vi "Start Live Mode.vi"(7 "Correlation ID":u32, 8 "error in (no error)":errorcluster, 9 "Mode":T1=enum."Live", 10 "Camera Settings":T2={"Exposure Time (ms)"=100.0, "Binning"=enum."2x2", "Scan Mode"=0, "Frames to Acquire"=1000.0, "Pixel Correction"=FALSE, "Frames to Skip"=0, "File Path"=path "", "Duty cycle"=0.0, "ALEX"=FALSE, "Shutter Enable"=[], "fluidics trigger, ms (0=disabled)"=0.0, "Bit Depth"=16, "Image Width (px)"=0, "Image Height (px)"=0, "Horizontal Offset (px)"=0, "Vertical Offset (px)"=0} {"fluidics trigger, ms (0=disabled)" max=60000.0 step=1.0; "Exposure Time (ms)" min=1.0 max=10000.0 step=1.0}, 11 "Application in":refnum<class "Application.lvclass">) -> (0 "error out":errorcluster, 3 "Application out":refnum<class "Application.lvclass">)   [LabVIEW 2023, in "Application.lvlib" / "Application.lvclass"]
uses:
  Application.lvclass
  Resources/Type Defs/Camera Settings.ctl
  Mode.ctl
  Application.lvclass/Application.ctl
  Hardware/Camera Messages/Start Live Mode Msg/Start Live Mode Msg.lvclass/Start Live Mode Msg.ctl
  <vilib>/ActorFramework/Message Enqueuer/Message Enqueuer.lvclass/Message Enqueuer.ctl
  Hardware/Sync Device Messages/Start Streaming Msg/Start Streaming Msg.lvclass/Start Streaming Msg.ctl
  <vilib>/ActorFramework/Message Enqueuer/Enqueue.vi
  Hardware/Camera Messages/Start Live Mode Msg/Start Live Mode Msg.lvclass
  Hardware/Sync Device Messages/Start Streaming Msg/Start Streaming Msg.lvclass
  Resources/GLOBAL/GLOBAL Time-critical.vi
  <vilib>/ActorFramework/Message Priority Queue/Priority Enqueue.vi
  Application.lvlib
  Hardware/NI DAQ/NI DAQ.lvlib
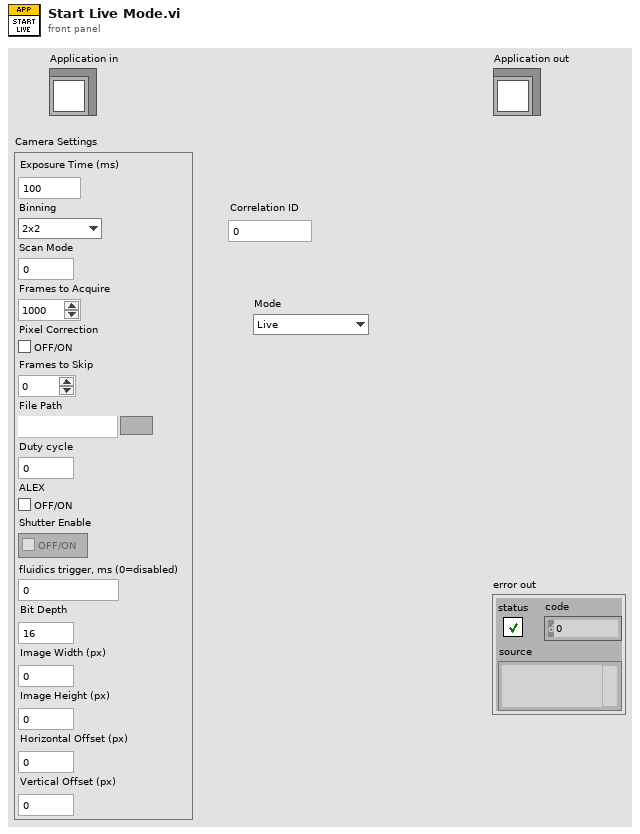
[diagram p1: front panel]
types:
  T1 = typedef "Application.lvlib/Mode.ctl" = enum16{"Idle", "Cancel", "Live", "Stream", "Autofocus", "Z-Stack", "Montage", "Saving", "Stage Scan", "Laser Adjust"}
  T2 = typedef "Camera Settings.ctl" = cluster{"Exposure Time (ms)":dbl, "Binning":enum16{"1x1", "2x2", "4x4"}, "Scan Mode":i32, "Frames to Acquire":dbl, "Pixel Correction":bool, "Frames to Skip":u32, "File Path":path, "Duty cycle":dbl, "ALEX":bool, "Shutter Enable":bool[], "fluidics trigger, ms (0=disabled)":dbl, "Bit Depth":u16, "Image Width (px)":u16, "Image Height (px)":u16, "Horizontal Offset (px)":u16, "Vertical Offset (px)":u16}
  T3 = typedef "Shutter Configuration.ctl" = cluster{"IO Line":tag, "Name":string, "Wavelength":u16, "Max rate (Hz)":dbl}
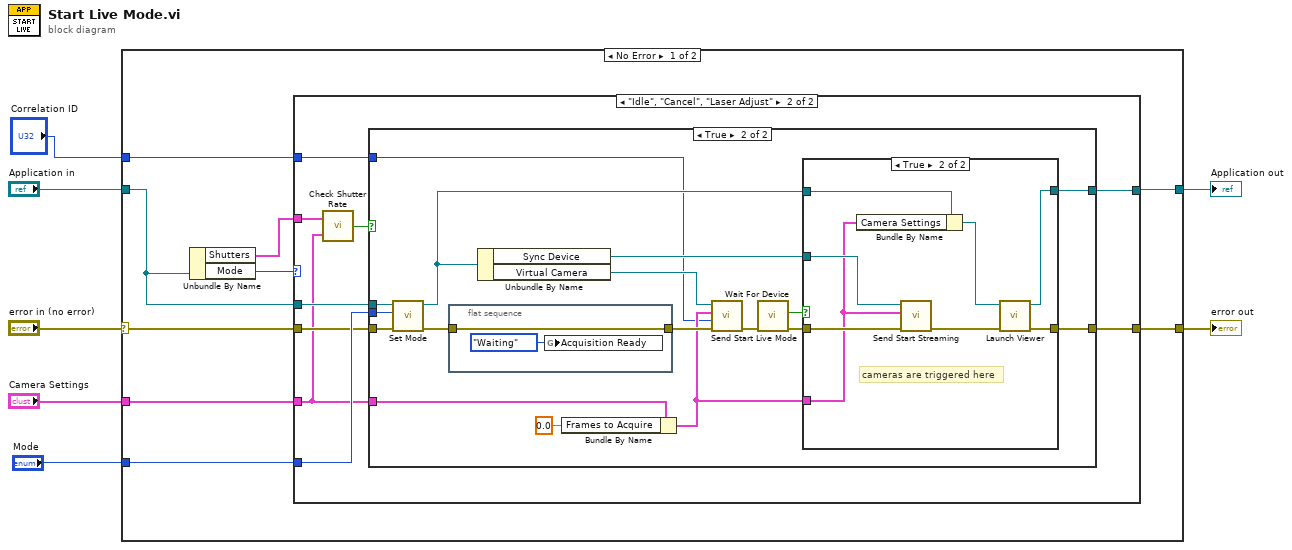
[diagram p0: block diagram]
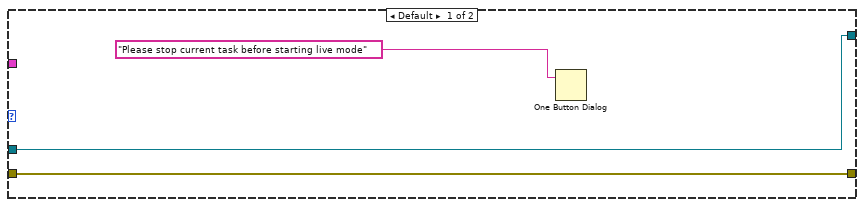
[diagram p2: hidden frame]
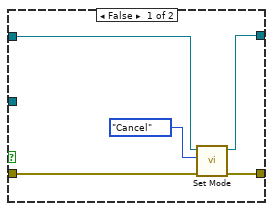
[diagram p4: hidden frame]
diagram:
  n1 = case shown="No Error" "error in (no error)" {
    selector: "error in (no error)" -> [w13 w64]
    tunnel: [w16 w64] -> w6
    tunnel: [w15 w63] -> w4
    tunnel: "Application in" -> [w12 w63]
    tunnel: "Camera Settings" -> [w14 _]
    tunnel: "Mode" -> [w10 _]
    tunnel: "Correlation ID" -> [w8 _]
    frame No Error {
      n2 = Unbundle By Name(w12) -> ("Shutters"=w9:T3[], "Mode"=w11:T1)
      n3 = case shown="\"Idle\", \"Cancel\", \"Laser Adjust\"" w11 {
        tunnel: [w18 w25] -> w16
        tunnel: [w19 w24] -> w15
        tunnel: w14 -> [_ w23]
        tunnel: w13 -> [w18 w27]
        tunnel: w12 -> [w19 w26]
        tunnel: w10 -> [_ w28]
        tunnel: w9 -> [_ w22]
        tunnel: w8 -> [_ w20]
        frame Default {
          n4 = One Button Dialog(message="Please stop current task before starting live mode") -> ()  [unwired: 1 in, 1 out]
        }
        frame "Idle", "Cancel", "Laser Adjust" {
          n5 = call "Check Shutter Rate.vi"("Camera Settings"=w23, "Shutters"=w22) -> ("OK?"=w21:bool)
          n6 = case shown="True" w21 {
            tunnel: w28 -> [_ w46]
            tunnel: w27 -> [w29 w45]
            tunnel: w26 -> [w30 w44]
            tunnel: [w29 w41] -> w25
            tunnel: [w30 w40] -> w24
            tunnel: w23 -> [_ w33]
            tunnel: w20 -> [_ w31]
            frame False {
            }
            frame True {
              n7 = call-dynamic "Set Mode.vi"("error in (no error)"=w45, "New Mode"=w46, "Application in"=w44) -> ("error out"=w43:errorcluster, "Application out"=w42:refnum<class "Application.lvclass">)  [unwired: 7 in]
              n8 = flat-sequence {
                tunnel: w43 -> [w62]
                tunnel: [w62] -> w39
                frame #0 {
                  n9 = global write "GLOBAL Time-critical.vi" "Acquisition Ready"(enum16{"Waiting", "Ready", "Fail", "Timeout"}."Waiting" ("Acquisition Ready")) -> ()
                }
              }
              n10 = Unbundle By Name(w42) -> ("Sync Device"=w47:refnum<class "Message Enqueuer.lvclass">, "Virtual Camera"=w38:refnum<class "Message Enqueuer.lvclass">)
              n11 = Bundle By Name(cluster=w33, "Frames to Acquire"=0.0) -> (w32:T2)
              n12 = call "Send Start Live Mode.vi"("error in (no error)"=w39, "Correlation ID"=w31, "Camera Settings"=w32, "Message Enqueuer"=w38) -> ("error out"=w37:errorcluster)  [unwired: 6 in, 1 out]
              n13 = call "Wait For Device.vi"("error in"=w37) -> ("error out"=w35:errorcluster, "Success?"=w36:bool)  [unwired: 9 in]
              n14 = case shown="True" w36 {
                tunnel: w47 -> [_ w54]
                tunnel: w42 -> [w51 w60]
                tunnel: [w49 w59] -> w41
                tunnel: [w50 w58] -> w40
                tunnel: w32 -> [_ w53]
                tunnel: w35 -> [w48 w55]
                frame False {
                  n15 = call-dynamic "Set Mode.vi"("error in (no error)"=w48, "New Mode"=Mode."Cancel", "Application in"=w51) -> ("error out"=w49:errorcluster, "Application out"=w50:refnum<class "Application.lvclass">)  [unwired: 7 in]
                }
                frame True {
                  # "cameras are triggered here"
                  n16 = Bundle By Name(cluster=w60, "Camera Settings"=w53) -> (w57:refnum<class "Application.lvclass">)
                  n17 = call "Send Start Streaming.vi"("error in (no error)"=w55, "Camera Settings"=w53, "Message Enqueuer"=w54) -> ("error out"=w56:errorcluster)  [unwired: 7 in, 1 out]
                  n18 = call-dynamic "Launch Viewer.vi"("error in (no error)"=w56, "Application in"=w57) -> ("error out"=w59:errorcluster, "Application out"=w58:refnum<class "Application.lvclass">)  [unwired: 8 in]
                }
              }
            }
          }
        }
      }
    }
    frame Error {
    }
  }
  "error out" <- w6
  "Application out" <- w4
